vi "Get Value (Value).vi"(8 "error in (no error)":errorcluster, 10 "key":string, 11 "JSON Value in":refnum<class "JSON Value.lvclass">) -> (0 "error out":errorcluster, 2 "JSON Value out":refnum<class "JSON Value.lvclass">)   [LabVIEW 2017, in "JSON Value.lvclass"]
uses:
  JSON Value.lvclass
  JSON Value.lvclass/JSON Value.ctl
  subVIs/Errors.ctl
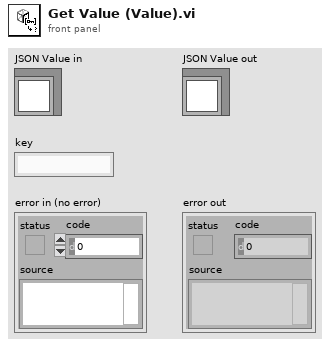
[diagram p1: front panel]
types:
  T1 = typedef "JSON Value.lvclass/Errors.ctl" = enum16{"No key", "Key path type", "Array OOB", "Type Mismatch", "Invalid Token"}
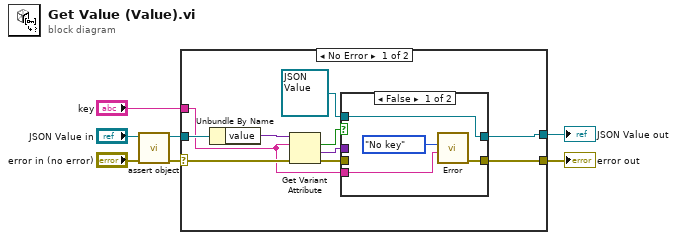
[diagram p0: block diagram]
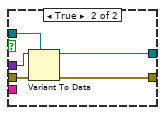
[diagram p2: hidden frame]
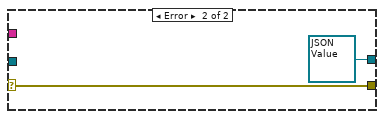
[diagram p3: hidden frame]
diagram:
  n1 = call "assert object.vi"("error in (no error)"="error in (no error)", "JSON Value in"="JSON Value in") -> ("error out"=w3:errorcluster, "JSON Value out"=w1:refnum<class "JSON Value.lvclass">)  [unwired: 8 in]
  n2 = case shown="No Error" w3 {
    selector: w3 -> [w15 w28]
    tunnel: [w13 w28] -> w6
    tunnel: w1 -> [w17 _]
    tunnel: "key" -> [w9 _]
    tunnel: [w12 refnum<class "JSON Value.lvclass"> refnum ("JSON Helper.lvclass")] -> w4
    frame No Error {
      n3 = Unbundle By Name(w17) -> ("value"=w11:variant)
      n4 = Get Variant Attribute(Variant=w11, name=w9, error in=w15) -> (found=w10:bool, value=w16:variant, error out=w14:errorcluster)  [unwired: 1 in, 1 out]
      n5 = case shown="False" w10 {
        tunnel: w16 -> [_ w26]
        tunnel: w14 -> [_ w25]
        tunnel: [w20 w24] -> w13
        tunnel: refnum<class "JSON Value.lvclass"> refnum ("JSON Helper.lvclass") -> [w21 w23]
        tunnel: [w21 w22] -> w12
        tunnel: w9 -> [w18 _]
        frame False {
          n6 = call "Error.vi"("Data"=w18, 9:Errors."No key") -> ("error out"=w20:errorcluster)  [unwired: 8 in]
        }
        frame True {
          n7 = Variant To Data(error in=w25, type=w23, Variant=w26) -> (data=w22:refnum<class "JSON Value.lvclass">, error out=w24:errorcluster)
        }
      }
    }
    frame Error {
    }
  }
  "error out" <- w6
  "JSON Value out" <- w4
